vi "test Import Configuration File.vi"(8 "error in":errorcluster, 11 "TestCase in":refnum<class "Import.lvclass">) -> (0 "error out":errorcluster, 3 "TestCase out":refnum<class "Import.lvclass">)   [LabVIEW 2020, in "Import.lvclass"]
uses:
  Import.lvclass
  <vilib>/addons/_JKI Toolkits/VI Tester/TestCase.llb/TestCase.lvclass
  Import/ARINC 429 Import.lvlib
  <vilib>/NI/VeriStand Custom Device Testing Tools/VeriStandTestUtilities/VeriStandTestUtilities.lvlib
  Shared/Transfer Type.ctl
  Shared/Direction.ctl
  Shared/Transfer Speed.ctl
  C:/Program Files (x86)/National Instruments/LabVIEW 2020/vi.lib/addons/_JKI Toolkits/VI Tester/TestCase.llb/TestCase.lvclass
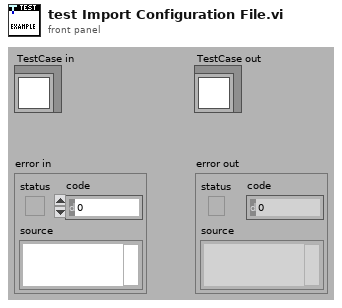
[diagram p1: front panel]
types:
  T1 = typedef "Direction.ctl" = enum16{"Rx", "Tx"}
  T2 = typedef "Transfer Type.ctl" = enum16{"Scheduled", "Acyclic", "Block", "Strobe"}
  T3 = typedef "Transfer Speed.ctl" = enum16{"LO (12.5 kb/s)", "HI (100 kb/s)"}
  T4 = cluster{"hardware channel":i32, "direction":T1, "labels":cluster{"label (Dec)":i32, "label (Display)":i32, "parameters":cluster{"name":string, "default value":dbl, "unit":string, "Parameter":cluster{"start index":i32, "size":i32, "encoding":enum16{"BNR", "BCD", "Discrete"}, "signed":bool, "scale multiplier":dbl, "scale offset":dbl}}[], "SDI value":u8, "SDI enabled":bool, "transfer type":T2, "SDI enabled 2":bool, "transmit period":u32}[], "speed":T3}[]
  T5 = typedef "VS Channels Definition for All Labels on Hardware Channel.ctl" = cluster{"hardware channel":i32, "direction":T1, "labels":T6[], "speed":T3}
  T6 = typedef "VS Channels Definition for Label.ctl" = cluster{"label (Dec)":u32, "label (Display)":u32, "parameters":T7[], "SDI value":u8, "SDI enabled":bool, "transfer type":T2, "create timestamp":bool, "transmit period":u32}
  T7 = typedef "VS Channel Definition for Parameter.ctl" = cluster{"name":string, "default value":dbl, "unit":string, "Parameter":T8}
  T8 = typedef "Parameter Definition.ctl" = cluster{"start index":i32, "size":i32, "encoding":T9, "signed":bool, "scale multiplier":dbl, "scale offset":dbl}
  T9 = typedef "Encoding and Decoding.lvlib/Encoding.ctl" = enum16{"BNR", "BCD", "Discrete"}
  T10 = cluster{"hardware channel":i32, "direction":T1, "labels":cluster{"label (Dec)":i32, "label (Display)":i32, "parameters":cluster{"name":string, "default value":dbl, "unit":string, "Parameter":cluster{"start index":i32, "size":i32, "encoding":enum16{"BNR", "BCD", "Discrete"}, "signed":bool, "scale multiplier":dbl, "scale offset":dbl}}[], "SDI value":u8, "SDI enabled":bool, "transfer type":T2, "SDI enabled 2":bool, "transmit period":u32}[], "speed":T3}
  T11 = cluster{"label (Dec)":i32, "label (Display)":i32, "parameters":cluster{"name":string, "default value":dbl, "unit":string, "Parameter":cluster{"start index":i32, "size":i32, "encoding":enum16{"BNR", "BCD", "Discrete"}, "signed":bool, "scale multiplier":dbl, "scale offset":dbl}}[], "SDI value":u8, "SDI enabled":bool, "transfer type":T2, "SDI enabled 2":bool, "transmit period":u32}[]
  T12 = cluster{"label (Dec)":i32, "label (Display)":i32, "parameters":cluster{"name":string, "default value":dbl, "unit":string, "Parameter":cluster{"start index":i32, "size":i32, "encoding":enum16{"BNR", "BCD", "Discrete"}, "signed":bool, "scale multiplier":dbl, "scale offset":dbl}}[], "SDI value":u8, "SDI enabled":bool, "transfer type":T2, "SDI enabled 2":bool, "transmit period":u32}
  T13 = cluster{"name":string, "default value":dbl, "unit":string, "Parameter":cluster{"start index":i32, "size":i32, "encoding":enum16{"BNR", "BCD", "Discrete"}, "signed":bool, "scale multiplier":dbl, "scale offset":dbl}}[]
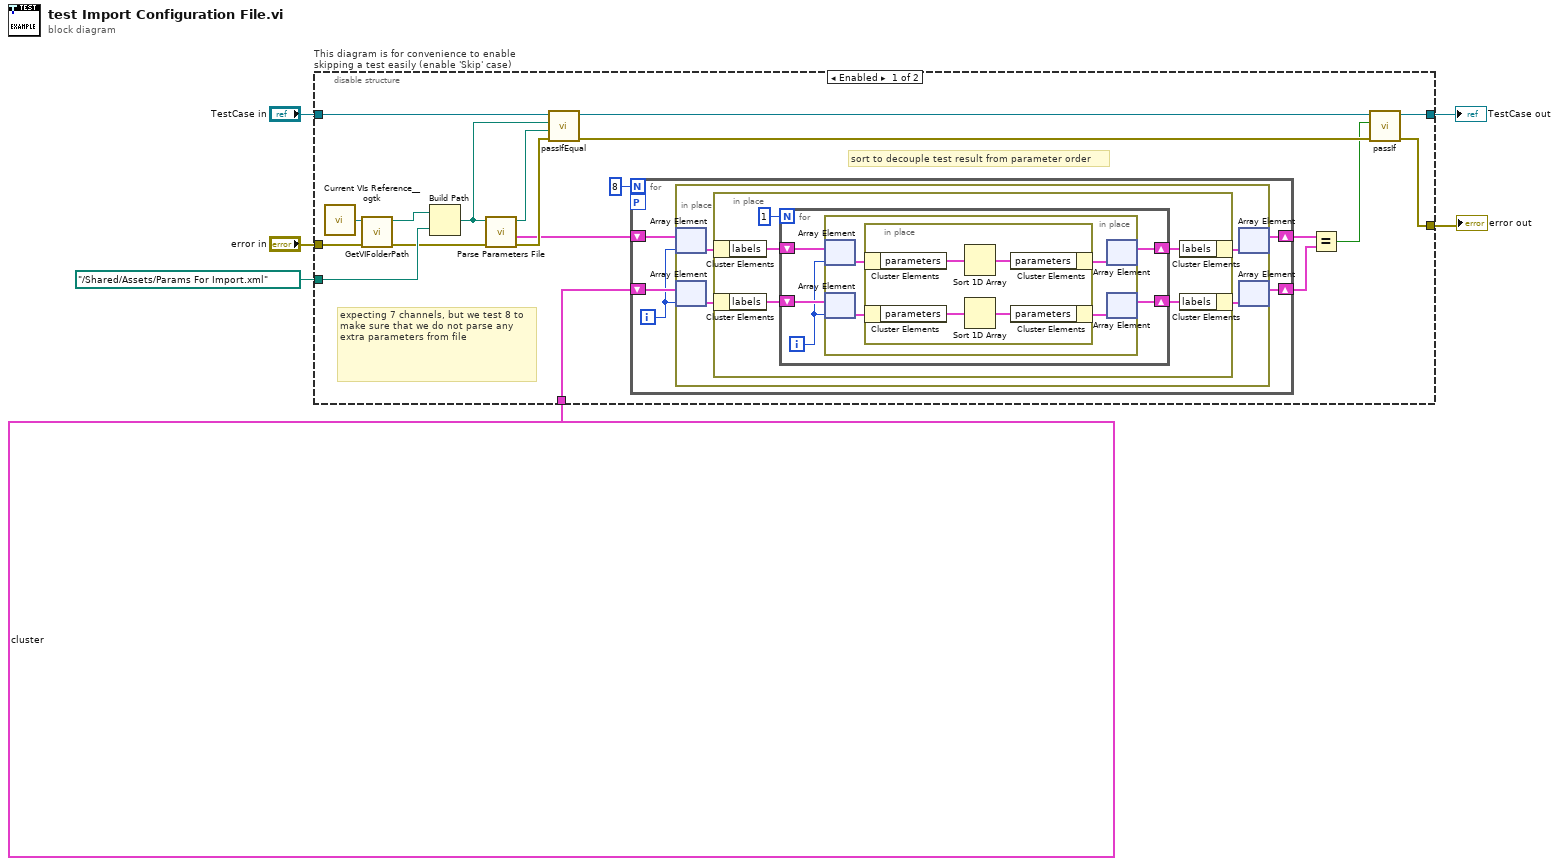
[diagram p0: block diagram]
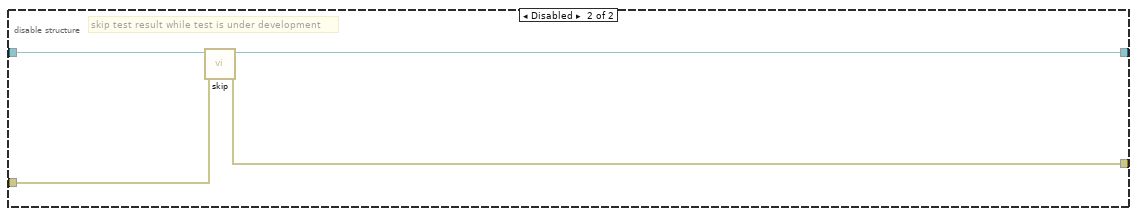
[diagram p2: hidden frame]
diagram:
  n1 = disable-structure "This diagram is for convenience to enable skipping a test easily (enable 'Skip' case)" shown="Enabled" {
    disable-tunnel: "TestCase in" -> [w25 w56]
    disable-tunnel: [w14 w54] -> w3
    disable-tunnel: [w15 w55] -> w5
    disable-tunnel: "error in" -> [w22 w53]
    disable-tunnel: path "../Shared/Assets/Params For Import.xml" ("Absolute or Relative Path") -> [w21 _]
    disable-tunnel: T4 [{"hardware channel"=0, "direction"=enum."Rx", "labels"=[{"label (Dec)"=134, "label (Display)"=134, "parameters"=[{"name"="Altitude_Rx", "default value"=0.0, "unit"="psi", "Parameter"={"start index"=18, "size"=10, "encoding"=enum."BNR", "signed"=TRUE, "scale multiplier"=16.0, "scale offset"=0.0}}, {"name"="SSM", "default value"=0.0, "unit"="", "Parameter"={"start index"=29, "size"=2, "encoding"=enum."BNR", "signed"=FALSE, "scale multiplier"=1.0, "scale offset"=0.0}}, {"name"="Parity", "default value"=0.0, "unit"="", "Parameter"={"start index"=31, "size"=1, "encoding"=enum."Discrete", "signed"=FALSE, "scale multiplier"=1.0, "scale offset"=0.0}}], "SDI value"=4, "SDI enabled"=FALSE, "transfer type"=enum."Scheduled", "SDI enabled 2"=TRUE, "transmit period"=0}], "speed"=enum."LO (12.5 kb/s)"}, {"hardware channel"=2, "direction"=enum."Rx", "labels"=[{"label (Dec)"=135, "label (Display)"=135, "parameters"=[{"name"="Altitude_Rx", "default value"=0.0, "unit"="ft", "Parameter"={"start index"=10, "size"=19, "encoding"=enum."BCD", "signed"=TRUE, "scale multiplier"=1.0, "scale offset"=0.0}}, {"name"="SSM", "default value"=0.0, "unit"="", "Parameter"={"start index"=29, "size"=2, "encoding"=enum."BNR", "signed"=FALSE, "scale multiplier"=1.0, "scale offset"=0.0}}], "SDI value"=4, "SDI enabled"=FALSE, "transfer type"=enum."Scheduled", "SDI enabled 2"=FALSE, "transmit period"=0}], "speed"=enum."HI (100 kb/s)"}, {"hardware channel"=4, "direction"=enum."Rx", "labels"=[{"label (Dec)"=136, "label (Display)"=136, "parameters"=[{"name"="Altitude_Rx", "default value"=0.0, "unit"="m", "Parameter"={"start index"=13, "size"=16, "encoding"=enum."BNR", "signed"=TRUE, "scale multiplier"=1.0, "scale offset"=0.0}}, {"name"="valid_Rx", "default value"=0.0, "unit"="", "Parameter"={"start index"=10, "size"=1, "encoding"=enum."Discrete", "signed"=FALSE, "scale multiplier"=1.0, "scale offset"=0.0}}, {"name"="current_Rx", "default value"=0.0, "unit"="", "Parameter"={"start index"=11, "size"=1, "encoding"=enum."Discrete", "signed"=FALSE, "scale multiplier"=1.0, "scale offset"=0.0}}, {"name"="SSM", "default value"=0.0, "unit"="", "Parameter"={"start index"=29, "size"=2, "encoding"=enum."BNR", "signed"=FALSE, "scale multiplier"=1.0, "scale offset"=0.0}}], "SDI value"=4, "SDI enabled"=FALSE, "transfer type"=enum."Scheduled", "SDI enabled 2"=FALSE, "transmit period"=0}], "speed"=enum."HI (100 kb/s)"}, {"hardware channel"=17, "direction"=enum."Tx", "labels"=[{"label (Dec)"=134, "label (Display)"=134, "parameters"=[{"name"="Altitude_Tx", "default value"=0.0, "unit"="psi", "Parameter"={"start index"=18, "size"=10, "encoding"=enum."BNR", "signed"=TRUE, "scale multiplier"=16.0, "scale offset"=0.0}}], "SDI value"=4, "SDI enabled"=FALSE, "transfer type"=enum."Scheduled", "SDI enabled 2"=FALSE, "transmit period"=20000}], "speed"=enum."HI (100 kb/s)"}, {"hardware channel"=19, "direction"=enum."Tx", "labels"=[{"label (Dec)"=135, "label (Display)"=135, "parameters"=[{"name"="Altitude_Tx", "default value"=0.0, "unit"="ft", "Parameter"={"start index"=10, "size"=19, "encoding"=enum."BCD", "signed"=TRUE, "scale multiplier"=1.0, "scale offset"=0.0}}], "SDI value"=4, "SDI enabled"=FALSE, "transfer type"=enum."Scheduled", "SDI enabled 2"=FALSE, "transmit period"=0}], "speed"=enum."HI (100 kb/s)"}, {"hardware channel"=21, "direction"=enum."Tx", "labels"=[{"label (Dec)"=136, "label (Display)"=136, "parameters"=[{"name"="Altitude_Tx", "default value"=0.0, "unit"="m", "Parameter"={"start index"=13, "size"=16, "encoding"=enum."BNR", "signed"=TRUE, "scale multiplier"=1.0, "scale offset"=0.0}}, {"name"="valid_Tx", "default value"=0.0, "unit"="", "Parameter"={"start index"=10, "size"=1, "encoding"=enum."Discrete", "signed"=FALSE, "scale multiplier"=1.0, "scale offset"=0.0}}, {"name"="current_Tx", "default value"=0.0, "unit"="", "Parameter"={"start index"=11, "size"=1, "encoding"=enum."Discrete", "signed"=FALSE, "scale multiplier"=1.0, "scale offset"=0.0}}], "SDI value"=4, "SDI enabled"=FALSE, "transfer type"=enum."Acyclic", "SDI enabled 2"=FALSE, "transmit period"=0}], "speed"=enum."LO (12.5 kb/s)"}] ("ports") -> [w10 _]
    frame Enabled {
      # "sort to decouple test result from parameter order"
      # "expecting 7 channels, but we test 8 to make sure that we do not parse any extra parameters from file"
      n2 = call <userlib>:"Current VIs Reference__ogtk.vi"() -> ("Current VI's reference"=w24:refnum<vi>)  [unwired: 5 in]
      n3 = call <vilib>:"GetVIFolderPath.vi"("error in (no error)"=w22, "VI Reference in"=w24) -> ("error out"=w19:errorcluster, "VI Folder Path out"=w23:path)  [unwired: 8 in]
      n4 = Build Path(base path=w23, name or relative path=w21) -> (appended path=w20:path)
      n5 = call "Parse Parameters File.vi"("error in"=w19, "path to XML document"=w20) -> ("error out"=w16:errorcluster, "ports"=w11:T5[], "path to XML document out"=w12:path)  [unwired: 7 in]
      n6 = call-dynamic "passIfEqual.vi"("error in (no error)"=w16, "y"=w12, "x"=w20, "TestCase in"=w25) -> ("error out"=w18:errorcluster, "TestCase out"=w17:refnum<class "Import.lvclass">)  [unwired: 6 in]
      n7 = for {
        N: 8 -> [_]
        shift-right: [w27] -> w9
        shift-left: w11 -> [w30]
        shift-right: [w26] -> w8
        shift-left: w10 -> [w29]
        workers-P: _ -> [_]
        i -> [w28]
        n8 = in-place {
          n9 = in-place-array #1(w30, w28) -> (w34:T5)
          n10 = in-place-array #2(w29, w28) -> (w33:T10)
          n11 = in-place {
            n12 = in-place-cluster #3(w34) -> ("labels"=w39:T6[])
            n13 = in-place-cluster #4(w33) -> ("labels"=w38:T11)
            n14 = for {
              N: 1 -> [_]
              shift-right: [w40] -> w37
              shift-left: w39 -> [w44]
              shift-right: [w41] -> w36
              shift-left: w38 -> [w43]
              i -> [w42]
              n15 = in-place {
                n16 = in-place-array #5(w44, w42) -> (w48:T6)
                n17 = in-place-array #6(w43, w42) -> (w47:T12)
                n18 = in-place {
                  n19 = in-place-cluster #7(w48) -> ("parameters"=w52:T7[])
                  n20 = in-place-cluster #8(w47) -> ("parameters"=w51:T13)
                  n21 = Sort 1D Array(array=w52) -> (sorted array=w50:T7[])
                  n22 = Sort 1D Array(array=w51) -> (sorted array=w49:T13)
                  n23 = in-place-cluster #7("parameters"=w50) -> (w46:T6)
                  n24 = in-place-cluster #8("parameters"=w49) -> (w45:T12)
                }
                n25 = in-place-array #5(w46) -> (w40:T6[])  [unwired: 1 out]
                n26 = in-place-array #6(w45) -> (w41:T11)  [unwired: 1 out]
              }
            }
            n27 = in-place-cluster #3("labels"=w37) -> (w32:T5)
            n28 = in-place-cluster #4("labels"=w36) -> (w31:T10)
          }
          n29 = in-place-array #1(w32) -> (w27:T5[])  [unwired: 1 out]
          n30 = in-place-array #2(w31) -> (w26:T4)  [unwired: 1 out]
        }
      }
      n31 = Equal?(x=w9, y=w8) -> (x = y?=w13:bool)
      n32 = call-dynamic "passIf.vi"("error in (no error)"=w18, "pass"=w13, "TestCase in"=w17) -> ("error out"=w15:errorcluster, "TestCase out"=w14:refnum<class "Import.lvclass">)  [unwired: 7 in]
    }
    frame Disabled {
      # "skip test result while test is under development"
      n33 = call <vilib>:"skip.vi"("error in (no error)"=w53, "TestCase in"=w56) -> ("error out"=w55:errorcluster, "TestCase out"=w54:refnum<class "Import.lvclass">)  [unwired: 8 in]
    }
  }
  "error out" <- w5
  "TestCase out" <- w3
